vi "Manual CV-K237_V1.2.vi"() -> ()   [LabVIEW 2009]
uses:
  <vilib>/xml/Close Reference(Node).vi
  subVIs/CMSFPIX_LV80.llb/Keith 237 Operate/Standby.vi
  <vilib>/Utility/file.llb/Write To Spreadsheet File (string).vi
  <vilib>/Utility/file.llb/Write To Spreadsheet File (DBL).vi
  <vilib>/xml/NI_XML.lvlib
panel:
  in  "Stop Loop":bool
  in  "Emergency Stop":bool
  in  "Set Lower Voltage Limit":i32=-1
  in  "Bias Loop":bool
  out "Bias":dbl=5.0
  out "Compliance Level":dbl
  out "Compliance":bool
  out "Compliance":dbl=1e-09
  out "Secondary Parameter":u16(ring) items=["None", "Cs", "Cp", "Ls", "Lp", "Rs", "Rp", "DF", "Q", "Z", "Y", "Phase", "ESR", "Gp", "Xs", "Bp"]
  out "Primary Parameter":u16(ring)=2 items=["AUTO", "Cs", "Cp", "Ls", "Lp", "Rs", "Rp", "DF", "Q", "Z", "Y", "Phase", "ESR", "Gp", "Xs", "Bp"]
  out "Voltage Level":dbl=0.15
  out "Secondary Graph":cluster{"Y":dbl[], "Y":dbl[]}[](graph) caption="DF"
  out "Number of Averages":dbl=1.0
  out "Frequency":dbl=1000.0
  out "Time Delay mS":dbl=1000.0
  in  "Voltage Start":dbl
  out "Running?":bool
  in  "Device ID":string
  in  "Halt Program":bool
  in  "error in (no error)":errorcluster
  out "error out":errorcluster
  in  "Voltage Steps":dbl=2.0
  in  "Set Upper Voltage Limit":i32=10
  out "Primary Graph":cluster{"Y":dbl[], "Y":dbl[]}[](graph) caption="Cp"
  out "Initialize":string
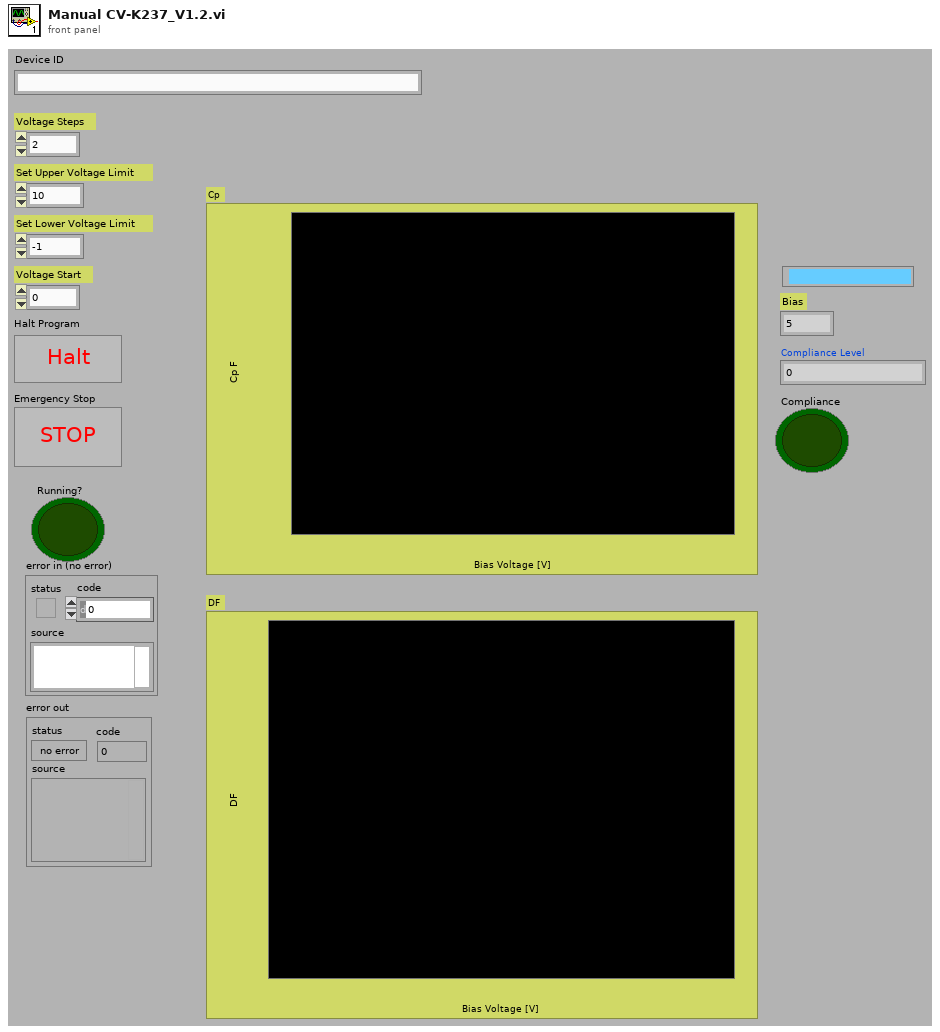
[diagram p1: front panel]
types:
  T1 = enum16{"open", "replace", "create", "open or create", "replace or create", "replace or create with confirmation"}
  T2 = cluster{"error":bool, "code":i32, "source":string}
  T3 = typedef "Semaphore RefNum" = refnum<k1>
  T4 = cluster{"error":bool, "code":i8, "source":string}
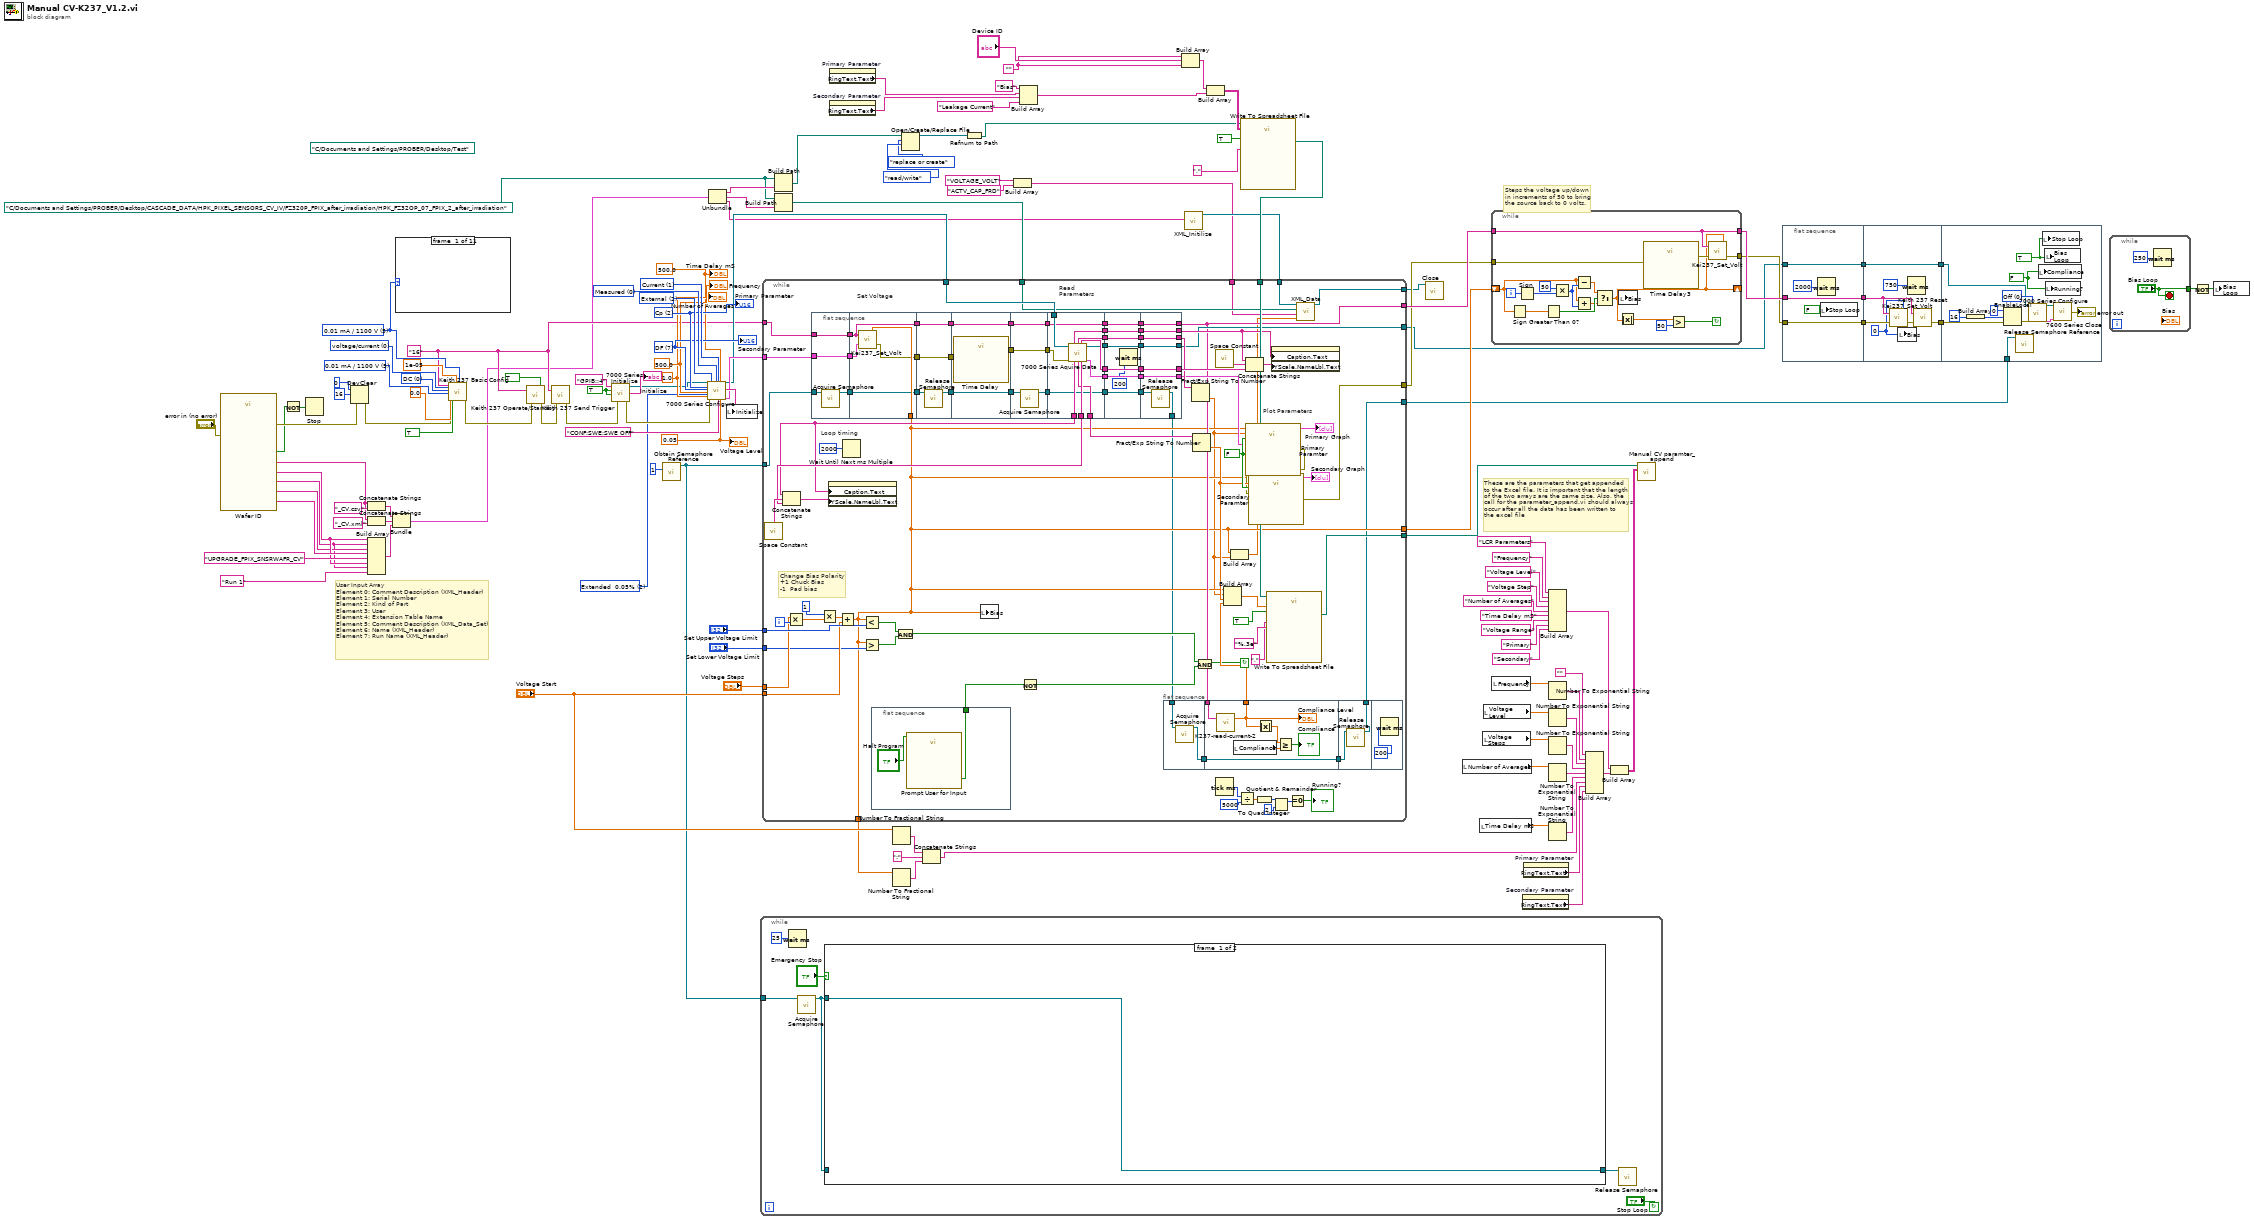
[diagram p0: block diagram]
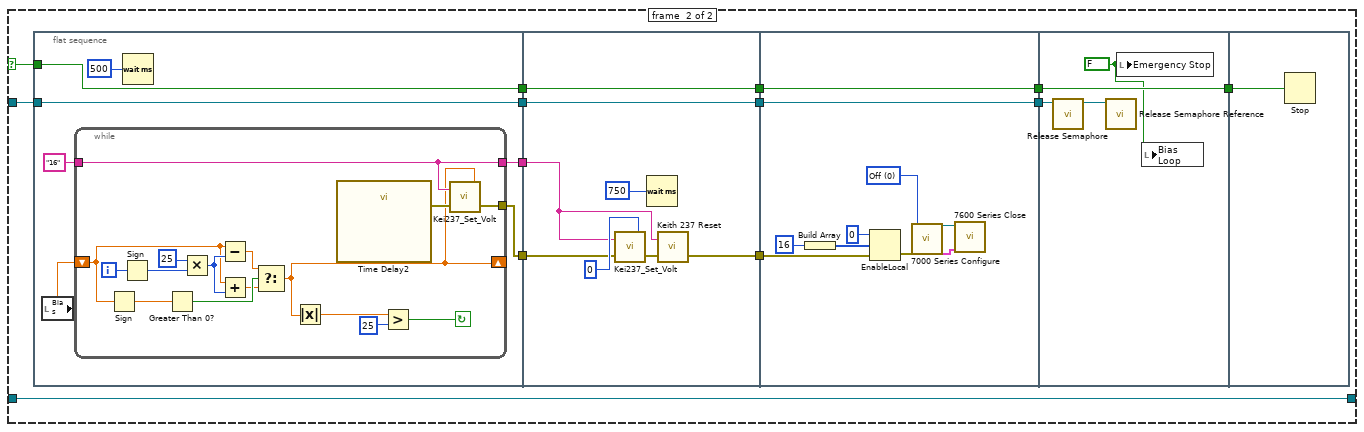
[diagram p2: hidden frame]
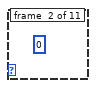
[diagram p3: hidden frame]
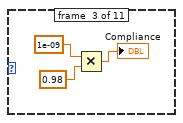
[diagram p4: hidden frame]
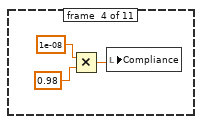
[diagram p5: hidden frame]
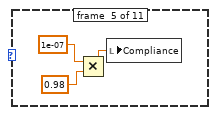
[diagram p6: hidden frame]
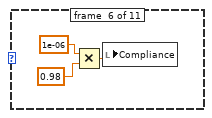
[diagram p7: hidden frame]
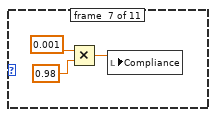
[diagram p8: hidden frame]
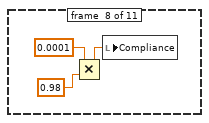
[diagram p9: hidden frame]
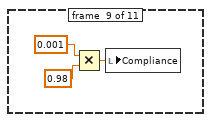
[diagram p10: hidden frame]
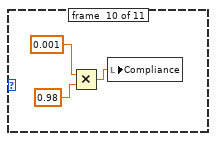
[diagram p11: hidden frame]
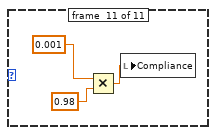
[diagram p12: hidden frame]
diagram:
  (unwired) path "C:/Documents and Settings/PROBER/Desktop/Test" ("base path")
  w87 = u16 2 items=["Basic        0.5%", "Enhanced 0.25%", "Extended  0.05%"] ("Measurement Accuracy")
  w70 = ""
  w19 = path "C:/Documents and Settings/PROBER/Desktop/CASCADE_DATA/HPK_PIXEL_SENSORS_CV_IV/FZ320P_FPIX_after_irradiation/HPK_FZ32OP_07_FPIX_2_after_irradiation" ("base path")
  w44 = u16 5 items=["auto / auto", "1 nA / 1.1 V", "10 nA / 11 V", "100 nA / 110 V", "0.001 mA / 1100 V", "0.01 mA / 1100 V", "0.1 mA / 1100 V", "1 mA / 1100 V", "10 mA / 1100 V", "100 mA / 1100 V"] ("compliance/\nmeasurement range (auto:0)")
  w107 = u16 5 items=["auto / auto", "1 nA / 1.1 V", "10 nA / 11 V", "100 nA / 110 V", "0.001 mA / 1100 V", "0.01 mA / 1100 V", "0.1 mA / 1100 V", "1 mA / 1100 V", "10 mA / 1100 V", "100 mA / 1100 V"] ("source range\nI source / V source (auto:0)")
  w112 = u16 0 items=["voltage/current", "current/voltage"] ("source/measure (V/I:0)")
  w113 = u16 0 items=["DC", "sweep"] ("function (DC:0)")
  w40 = "16" ("GPIB address")
  w115 = 500.0 ("Time Delay mS")
  w117 = TRUE ("reset")
  w69 = 0.05 ("Voltage Level")
  w122 = 1.0 ("Number of Averages")
  w123 = 500.0 ("Frequency")
  w124 = u16 7 items=["None", "Cs", "Cp", "Ls", "Lp", "Rs", "Rp", "DF", "Q", "Z", "Y", "Phase", "ESR", "Gp", "Xs", "Bp"] ("Secondary Parameter")
  w125 = u16 2 items=["AUTO", "Cs", "Cp", "Ls", "Lp", "Rs", "Rp", "DF", "Q", "Z", "Y", "Phase", "ESR", "Gp", "Xs", "Bp"] ("Primary Parameter")
  w126 = u16 1 items=["Voltage", "Current"] ("Signal Type")
  w127 = u16 0 items=["Measured", "Deviation", "% Deviation", "No Display"] ("Display")
  w128 = u16 2 items=["Off", "Internal", "External"] ("Bias")
  # "User Input Array\nElement 0: Comment Description (XML_Header)\nElement 1: Serial Number\nElement 2: Kind of Part\nElement 3: User\nElement 4: Extension Table Name\nElement 5: Comment Description (XML_Data_Set)\nElement 6: Name (XML_Header)\nElement 7: Run Name (XML_Header)"
  # "These are the parameters that get appended\nto the Excel file. It is important that the length\nof the two arrays are the same size. Also, the\ncall for the parameter_append.vi should always\noccur after all the data has been written to\nthe excel file"
  # "Steps the voltage up/down\nin increments of 50 to bring\nthe source back to 0 volts."
  n1 = call "Wafer ID"("error in (no error)"="error in (no error)") -> ("Test Name"=w7:string, "User"=w6:string, "Kind of Part"=w3:string, "Part Name"=w2:string, "Comment Description"=w4:string, "OK"=w93:bool, "error out"=w98:errorcluster)  [unwired: 11 in, 1 out]
  n2 = Not(x=w93) -> (.not. x?=w92:bool)
  n3 = Stop(stop? (T)=w92) -> ()
  n4 = DevClear(2:w98, 3:i16 16 ("address"), 4:0) -> (0:w103:errorcluster)  [unwired: 1 out]
  n5 = Concatenate Strings(w7, "_CV.csv" ("string")) -> (w24:string)
  n6 = Concatenate Strings(w7, "_CV.xml" ("string")) -> (w23:string)
  n7 = Build Array(w4, w2, w3, w6, "UPGRADE_FPIX_SNSRWAFR_CV", w4, w2, "Run 1" ("element")) -> (w13:string[])
  n8 = Bundle(w24, w23, w13) -> (w20:cluster{string, string, string[]})  [unwired: 1 in]
  n9 = case shown="1" w44 {
    frame #0 {
    }
    frame #1 {
      (unwired) 0
    }
    frame #2 {
      n10 = Multiply(x=1e-09, y=0.98) -> (x*y=→"Compliance":dbl)
    }
    frame #3 {
      n11 = Multiply(x=1e-08, y=0.98) -> (x*y=w133:dbl)
      n12 = local write "Compliance"(w133) -> ()
    }
    frame #4 {
      n13 = Multiply(x=1e-07, y=0.98) -> (x*y=w136:dbl)
      n14 = local write "Compliance"(w136) -> ()
    }
    frame #5 {
      n15 = Multiply(x=1e-06, y=0.98) -> (x*y=w139:dbl)
      n16 = local write "Compliance"(w139) -> ()
    }
    frame #6 {
      n17 = Multiply(x=0.001, y=0.98) -> (x*y=w143:dbl)
      n18 = local write "Compliance"(w143) -> ()
    }
    frame #7 {
      n19 = Multiply(x=0.0001, y=0.98) -> (x*y=w145:dbl)
      n20 = local write "Compliance"(w145) -> ()
    }
    frame #8 {
      n21 = Multiply(x=0.001, y=0.98) -> (x*y=w149:dbl)
      n22 = local write "Compliance"(w149) -> ()
    }
    frame #9 {
      n23 = Multiply(x=0.001, y=0.98) -> (x*y=w151:dbl)
      n24 = local write "Compliance"(w151) -> ()
    }
    frame #10 {
      n25 = Multiply(x=0.001, y=0.98) -> (x*y=w154:dbl)
      n26 = local write "Compliance"(w154) -> ()
    }
  }
  n27 = call "Keith 237 Basic Config.vi"("GPIB address"=w40, "source/measure (V/I:0)"=w112, "function (DC:0)"=w113, "source range\nI source / V source (auto:0)"=w107, "source level"=0.0, "error in"=w103, "1100 V range (disabled:F)"=TRUE, "current \ncompliance level"=1e-05 ("current \ncompliance level"), "compliance/\nmeasurement range (auto:0)"=w44) -> ("error out"=w110:T2)  [unwired: 10 in]
  n28 = call "Keith 237 Operate/Standby.vi"("source"=TRUE, "error in"=w110, "GPIB address"=w40) -> ("error out"=w108:T2)
  n29 = call "Keith 237 Send Trigger.vi"("GPIB address"=w40, "error in"=w108) -> ("error out"=w102:T2)
  n30 = call "7000 Series Initialize.vi"("error in (no error)"=w102, "reset"=w117, "ID query"=w117, "instrument descriptor"="GPIB::4") -> ("error out"=w129:errorcluster, "Identification"=→"Initialize":string, "VISA session"=w118:refnum<visa-resource-name>)
  n31 = call <vilib>:"Obtain Semaphore Reference.vi"("size (1)"=1) -> ("semaphore"=w10:T3)  [unwired: 4 in, 2 out]
  n32 = call "7000 Series Configure.vi"("inst handle in"=w118, "Primary Parameter"=w125, "Secondary Parameter"=w124, "Frequency"=w123, "Measurement Accuracy"=w87, "Number of Averages"=w122, "error in"=w129, "Bias"=w128, "Display"=w127, "Signal Type"=w126, "Optional"="CONF:SWE:SWE OFF", "Time Delay mS"=w115, "Voltage Level"=w69) -> ("inst handle out"=w100:refnum<visa-resource-name>, "Identification"=w119:string, "error out"=w101:T4)  [unwired: 12 in]
  n33 = Unbundle(w20) -> (w22:string, w21:string, w12:string[])
  n34 = local write "Initialize"(w119) -> ()
  n35 = while {
    tunnel: w10 -> [w161]
    stop <- "Stop Loop" continue-if-true
    n36 = Wait (ms)(milliseconds to wait=25) -> ()  [unwired: 1 out]
    n37 = call <vilib>:"Acquire Semaphore.vi"("semaphore"=w161) -> ("semaphore out"=w158:T3)  [unwired: 4 in, 2 out]
    n38 = case shown="True" "Emergency Stop" {
      selector: "Emergency Stop" -> [_ w175]
      tunnel: w158 -> [w163 w176]
      tunnel: [w163 w173] -> w159
      tunnel: w158 -> [_ w173]
      frame #0 {
      }
      frame #1 {
        n39 = flat-sequence {
          tunnel: [w182] -> w172
          tunnel: w176 -> [w182]
          tunnel: [w181] -> w171
          tunnel: w175 -> [w181]
          tunnel: [w180] -> w166
          tunnel: [w178] -> w165
          tunnel: w172 -> [w207]
          tunnel: [w207] -> w170
          tunnel: w171 -> [w206]
          tunnel: [w206] -> w168
          tunnel: w166 -> [w202]
          tunnel: w165 -> [w201]
          tunnel: [w200] -> w164
          tunnel: w170 -> [w217]
          tunnel: [w217] -> w169
          tunnel: w168 -> [w216]
          tunnel: [w216] -> w167
          tunnel: w164 -> [w208]
          tunnel: w169 -> [w219]
          tunnel: w167 -> [w221]
          tunnel: [w221] -> w174
          tunnel: w174 -> [w222]
          frame #0 {
            n40 = local read "Bias"() -> (w177:dbl)
            n41 = while {
              tunnel: [w199] -> w180
              tunnel: "16" ("GPIB address") -> [w194]
              tunnel: [w194] -> w178
              shift-right: [w184] -> _
              shift-left: w177 -> [w187]
              i -> [w186]
              stop <- w196 continue-if-true
              n42 = Sign(1:w187) -> (0:w193:dbl)
              n43 = Sign(1:w186) -> (0:w185:i32)
              n44 = Greater Than 0?(x=w193) -> (x > 0?=w192:bool)
              n45 = Multiply(x=25, y=w185) -> (x*y=w191:i32)
              n46 = Subtract(x=w187, y=w191) -> (x-y=w190:dbl)
              n47 = Add(x=w187, y=w191) -> (x+y=w189:dbl)
              n48 = Select(t=w190, s=w192, f=w189) -> (s? t:f=w184:dbl)
              n49 = Absolute Value(x=w184) -> (abs(x)=w188:dbl)
              n50 = call "Time Delay2"() -> ("error out"=w195:errorcluster)  [unwired: 11 in]
              n51 = Greater?(x=w188, y=25) -> (0:w196:bool)
              n52 = call "Kei237_Set_Volt.vi"("Voltage"=w184, "error in"=w195, "GPIB"=w194) -> ("error out"=w199:errorcluster)
            }
            n53 = Wait (ms)(milliseconds to wait=500) -> ()  [unwired: 1 out]
          }
          frame #1 {
            n54 = call "Kei237_Set_Volt.vi"("Voltage"=0, "error in"=w202, "GPIB"=w201) -> ("error out"=w203:errorcluster)
            n55 = Wait (ms)(milliseconds to wait=750) -> ()  [unwired: 1 out]
            n56 = call "Keith 237 Reset.vi"("GPIB address"=w201, "error in"=w203) -> ("error out"=w200:T2)
          }
          frame #2 {
            w214 = u16 0 items=["Off", "Internal", "External"] ("Bias")
            n57 = Build Array(16) -> (w215:i32[])
            n58 = EnableLocal(2:w208, 3:w215, 4:0) -> (0:w211:errorcluster)  [unwired: 1 out]
            n59 = call "7000 Series Configure.vi"("error in"=w211, "Bias"=w214) -> ("inst handle out"=w212:refnum<visa-resource-name>, "error out"=w213:T4)  [unwired: 23 in, 1 out]
            n60 = call "7600 Series Close.vi"("error in (no error)"=w213, "VISA session"=w212) -> ()  [unwired: 2 in, 1 out]
          }
          frame #3 {
            w220 = FALSE ("Emergency Stop")
            n61 = call <vilib>:"Release Semaphore.vi"("semaphore"=w219) -> ("semaphore out"=w218:T3)  [unwired: 5 in, 1 out]
            n62 = call <vilib>:"Release Semaphore Reference.vi"("semaphore"=w218) -> ()  [unwired: 9 in, 2 out]
            n63 = local write "Emergency Stop"(w220) -> ()
            n64 = local write "Bias Loop"(w220) -> ()
          }
          frame #4 {
            n65 = Stop(stop? (T)=w222) -> ()
          }
        }
      }
    }
    n66 = call <vilib>:"Release Semaphore.vi"("semaphore"=w159) -> ()  [unwired: 5 in, 2 out]
  }
  n67 = Build Path(base path=w19, name or relative path=w22) -> (appended path=w85:path)
  n68 = Build Path(base path=w19, name or relative path=w21) -> (appended path=w17:path)
  n69 = property on="Secondary Parameter" class="Ring (strict)"() -> ("RingText.Text"=w51:string)  [unwired: 2 in, 2 out]
  n70 = property on="Primary Parameter" class="Ring (strict)"() -> ("RingText.Text"=w52:string)  [unwired: 2 in, 2 out]
  n71 = Number To Fractional String(number="Voltage Start") -> (F-format string=w45:string)  [unwired: 3 in]
  n72 = Open/Create/Replace File(file path (use dialog)=w85, operation (0:open)=T1."replace or create", access (0:read/write)=enum16{"read/write", "read-only", "write-only"}."read/write") -> (refnum out=w80:refnum<file>)  [unwired: 1 in, 4 out]
  n73 = Refnum to Path(1:w80) -> (0:w79:path)
  n74 = Build Array("VOLTAGE_VOLT", "ACTV_CAP_FRD") -> (w14:string[])
  n75 = Build Array("Bias", w52, w51, "Leakage Current" ("element")) -> (w90:string[])
  n76 = Build Array(w70, "Device ID", w70) -> (w89:string[])
  n77 = call "XML_Initilize.vi"("User Input"=w12) -> ("DOM document out"=w18:refnum<k20>)  [unwired: 10 in]
  n78 = Build Array(w89, w90) -> (w88:string[][])
  n79 = call-poly <vilib>:"Write To Spreadsheet File.vi"("delimiter (\\t)"=",", "append to file? (new file:F)"=TRUE, "2D data"=w88, "file path (dialog if empty)"=w79) -> ("new file path (Not A Path if cancelled)"=w78:path)  [unwired: 3 in, 1 out]
  n80 = while {
    tunnel: w40 -> [w285]
    tunnel: w101 -> [w284]
    tunnel: "Set Upper Voltage Limit" -> [w299]
    tunnel: "Voltage Steps" -> [w288]
    tunnel: w100 -> [w283]
    tunnel: [w287] -> w37
    tunnel: w78 -> [w309]
    tunnel: [w274] -> w39
    tunnel: "Voltage Start" -> [w289]
    tunnel: [w290] -> w73
    tunnel: [w255] -> w47
    tunnel: [w255] -> w38
    tunnel: [w275] -> w32
    tunnel: "Set Lower Voltage Limit" -> [w259]
    tunnel: w18 -> [w258]
    tunnel: w17 -> [w257]
    tunnel: w14 -> [w256]
    tunnel: w10 -> [w228]
    tunnel: [w224] -> w9
    tunnel: [w223] -> w8
    i -> [w314]
    stop <- w265 continue-if-true
    w296 = FALSE ("Reset")
    # "Read \nParameters"
    # "Set Voltage"
    # "Change Bias Polarity\n+1 Chuck Bias\n-1  Pad bias"
    # "Loop timing"
    # "Plot Parameters"
    n81 = call <vilib>:"Space Constant.vi"() -> ("String"=w292:string)
    n82 = Concatenate Strings(w276, w292, w278) -> (w291:string)
    n83 = Multiply(x=w288, y=w314) -> (x*y=w312:dbl)
    n84 = flat-sequence {
      tunnel: w285 -> [w328]
      tunnel: w284 -> [w329]
      tunnel: [w329] -> w237
      tunnel: [w328] -> w236
      tunnel: [w327] -> w234
      tunnel: w228 -> [w326]
      tunnel: w255 -> [w333]
      tunnel: [w332] -> w241
      tunnel: [w331] -> w239
      tunnel: w237 -> [w334]
      tunnel: w236 -> [w331]
      tunnel: [w330] -> w235
      tunnel: w234 -> [w330]
      tunnel: w241 -> [w338]
      tunnel: [w338] -> w240
      tunnel: w239 -> [w337]
      tunnel: [w337] -> w238
      tunnel: w235 -> [w336]
      tunnel: [w335] -> w232
      tunnel: w240 -> [w342]
      tunnel: [w341] -> w245
      tunnel: [w340] -> w243
      tunnel: w238 -> [w340]
      tunnel: [w339] -> w233
      tunnel: w232 -> [w339]
      tunnel: w245 -> [w346]
      tunnel: [w346] -> w244
      tunnel: w243 -> [w345]
      tunnel: [w345] -> w242
      tunnel: w233 -> [w344]
      tunnel: [w343] -> w229
      tunnel: w244 -> [w358]
      tunnel: w283 -> [w357]
      tunnel: [w352] -> w276
      tunnel: [w351] -> w278
      tunnel: [w350] -> w277
      tunnel: w242 -> [w348]
      tunnel: [w356] -> w272
      tunnel: [w355] -> w271
      tunnel: [w354] -> w270
      tunnel: [w353] -> w269
      tunnel: [w349] -> w268
      tunnel: [w348] -> w267
      tunnel: [w347] -> w230
      tunnel: w229 -> [w347]
      tunnel: w272 -> [w366]
      tunnel: w271 -> [w365]
      tunnel: w270 -> [w364]
      tunnel: w269 -> [w363]
      tunnel: w268 -> [w362]
      tunnel: w267 -> [w361]
      tunnel: [w366] -> w251
      tunnel: [w365] -> w250
      tunnel: [w364] -> w249
      tunnel: [w363] -> w248
      tunnel: [w362] -> w247
      tunnel: [w361] -> w246
      tunnel: [w359] -> w231
      tunnel: w230 -> [w359]
      tunnel: [w369] -> w274
      tunnel: [w370] -> w275
      tunnel: [w371] -> w279
      tunnel: [w372] -> w280
      tunnel: [w373] -> w282
      tunnel: [w374] -> w281
      tunnel: w251 -> [w374]
      tunnel: w250 -> [w373]
      tunnel: w249 -> [w372]
      tunnel: w248 -> [w371]
      tunnel: w247 -> [w370]
      tunnel: w246 -> [w369]
      tunnel: w231 -> [w368]
      tunnel: [w367] -> w227
      frame #0 {
        n85 = call <vilib>:"Acquire Semaphore.vi"("semaphore"=w326) -> ("semaphore out"=w327:T3)  [unwired: 4 in, 2 out]
      }
      frame #1 {
        n86 = call "Kei237_Set_Volt.vi"("Voltage"=w333, "error in"=w334, "GPIB"=w331) -> ("error out"=w332:errorcluster)
      }
      frame #2 {
        n87 = call <vilib>:"Release Semaphore.vi"("semaphore"=w336) -> ("semaphore out"=w335:T3)  [unwired: 5 in, 1 out]
      }
      frame #3 {
        n88 = call "Time Delay"("error in (no error)"=w342) -> ("error out"=w341:errorcluster)  [unwired: 10 in]
      }
      frame #4 {
        n89 = call <vilib>:"Acquire Semaphore.vi"("semaphore"=w344) -> ("semaphore out"=w343:T3)  [unwired: 4 in, 2 out]
      }
      frame #5 {
        n90 = call "7000 Series Aquire Data.vi"("inst handle in"=w357, "error in"=w358) -> ("Primary"=w356:string, "Primary Value"=w354:string, "Primary Unit"=w355:string, "inst handle out"=w349:refnum<visa-resource-name>, "Secondary"=w352:string, "Secondary Value"=w350:string, "Secondary Unit"=w351:string, "error out"=w353:T4)  [unwired: 5 in, 1 out]
      }
      frame #6 {
        n91 = Wait (ms)(milliseconds to wait=200) -> ()  [unwired: 1 out]
      }
      frame #7 {
        n92 = call <vilib>:"Release Semaphore.vi"("semaphore"=w368) -> ("semaphore out"=w367:T3)  [unwired: 5 in, 1 out]
      }
    }
    n93 = Multiply(x=1, y=w312) -> (x*y=w300:dbl)
    n94 = property on="Secondary Parameter" class="XYGraph (strict)"("Caption.Text"=w276, "YScale.NameLbl.Text"=w291) -> ()  [unwired: 2 in, 2 out]
    n95 = Add(x=w300, y=w289) -> (x+y=w255:dbl)
    n96 = Wait Until Next ms Multiple(millisecond multiple=u32 2000) -> ()  [unwired: 1 out]
    n97 = Less?(x=w255, y=w299) -> (x < y?=w262:bool)
    n98 = Greater?(x=w255, y=w259) -> (0:w261:bool)
    n99 = flat-sequence {
      tunnel: [w375] -> w263
      frame #0 {
        n100 = call "Prompt User for Input"("Enable"="Halt Program") -> ("Yes"=w375:bool)  [unwired: 17 in, 1 out]
      }
    }
    n101 = And(x=w262, y=w261) -> (x .and. y?=w260:bool)
    n102 = local write "Bias"(w255) -> ()
    n103 = Not(x=w263) -> (.not. x?=w264:bool)
    n104 = flat-sequence {
      tunnel: w227 -> [w316]
      tunnel: [w315] -> w225
      tunnel: w274 -> [w320]
      tunnel: [w318] -> w266
      tunnel: [w317] -> w226
      tunnel: w225 -> [w317]
      tunnel: w226 -> [w324]
      tunnel: [w323] -> w223
      frame #0 {
        n105 = call <vilib>:"Acquire Semaphore.vi"("semaphore"=w316) -> ("semaphore out"=w315:T3)  [unwired: 4 in, 2 out]
      }
      frame #1 {
        n106 = call "K237-read-current-2.vi"("GPIB"=w320) -> ("Current"=w318:dbl)  [unwired: 1 in, 1 out]
        "Compliance Level" <- w318
        n107 = local read "Compliance"() -> (w322:dbl)
        n108 = Absolute Value(x=w318) -> (abs(x)=w319:dbl)
        n109 = Greater Or Equal?(x=w319, y=w322) -> (x >= y?=→"Compliance":bool)
      }
      frame #2 {
        n110 = call <vilib>:"Release Semaphore.vi"("semaphore"=w324) -> ("semaphore out"=w323:T3)  [unwired: 5 in, 1 out]
      }
      frame #3 {
        n111 = Wait (ms)(milliseconds to wait=200) -> ()  [unwired: 1 out]
      }
    }
    n112 = Fract/Exp String To Number(string=w280) -> (number=w254:dbl)  [unwired: 3 in, 1 out]
    n113 = Fract/Exp String To Number(string=w277) -> (number=w295:dbl)  [unwired: 3 in, 1 out]
    n114 = And(x=w260, y=w264) -> (x .and. y?=w265:bool)
    n115 = Tick Count (ms)() -> (millisecond timer value=w305:u32)
    n116 = call <vilib>:"Space Constant.vi"() -> ("String"=w293:string)
    n117 = Build Array(w255, w254, w295, w266) -> (w253:dbl[])
    n118 = Build Array(w255, w254) -> (w252:dbl[])
    n119 = Divide(x=w305, y=5000) -> (x/y=w303:dbl)
    n120 = call "Primary Paramter"("error in (no error)"=w279, "Reset"=w296, "Y Input"=w254, "X Input"=w255) -> ("error out"=w286:errorcluster, "XY Graph"=→"Primary Graph":cluster{"Y":dbl[], "Y":dbl[]}[])  [unwired: 1 in, 5 out]
    n121 = Concatenate Strings(w281, w293, w282) -> (w294:string)
    n122 = call "Secondary Paramter"("error in (no error)"=w286, "Reset"=w296, "Y Input"=w295, "X Input"=w255) -> ("error out"=w287:errorcluster, "XY Graph"=→"Secondary Graph":cluster{"Y":dbl[], "Y":dbl[]}[])  [unwired: 1 in, 5 out]
    n123 = To Quad Integer(1:w303) -> (0:w302:i64)
    n124 = call-poly <vilib>:"Write To Spreadsheet File.vi"("delimiter (\\t)"=",", "format (%.3f)"="%.3e" ("file format"), "append to file? (new file:F)"=TRUE, "1D data"=w253, "file path (dialog if empty)"=w309) -> ("new file path (Not A Path if cancelled)"=w290:path)  [unwired: 2 in, 1 out]
    n125 = property on="Primary Parameter" class="XYGraph (strict)"("Caption.Text"=w281, "YScale.NameLbl.Text"=w294) -> ()  [unwired: 2 in, 2 out]
    n126 = Quotient & Remainder(x=w302, y=2) -> (x-y*floor(x/y)=w306:i64)  [unwired: 1 out]
    n127 = Equal To 0?(x=w306) -> (x = 0?=→"Running?":bool)
    n128 = call "XML_Data.vi"("Data Input Array"=w252, "Data Tag Names Array"=w256, "XML File Path"=w257, "DOM document in"=w258) -> ("DOM document out"=w224:refnum<k20>)  [unwired: 6 in, 1 out]
  }
  n129 = Number To Fractional String(number=w47) -> (F-format string=w49:string)  [unwired: 3 in]
  n130 = Concatenate Strings(w45, ":", w49) -> (w46:string)
  n131 = call-poly <vilib>:"Close.vi"("node"=w9) -> ()  [unwired: 8 in, 1 out]
  n132 = local read "Number of Averages"() -> (w82:dbl)
  n133 = local read "Time Delay mS"() -> (w81:dbl)
  n134 = local read "Voltage Steps"() -> (w83:dbl)
  n135 = local read "Voltage Level"() -> (w68:dbl)
  n136 = while {
    tunnel: [w393] -> w35
    tunnel: w37 -> [w388]
    tunnel: w39 -> [w387]
    tunnel: [w387] -> w36
    shift-right: [w377] -> _
    shift-left: w38 -> [w380]
    i -> [w379]
    stop <- w390 continue-if-true
    n137 = Sign(1:w380) -> (0:w386:dbl)
    n138 = Sign(1:w379) -> (0:w378:i32)
    n139 = Greater Than 0?(x=w386) -> (x > 0?=w385:bool)
    n140 = Multiply(x=50, y=w378) -> (x*y=w384:i32)
    n141 = Subtract(x=w380, y=w384) -> (x-y=w383:dbl)
    n142 = Add(x=w380, y=w384) -> (x+y=w382:dbl)
    n143 = Select(t=w383, s=w385, f=w382) -> (s? t:f=w377:dbl)
    n144 = local write "Bias"(w377) -> ()
    n145 = Absolute Value(x=w377) -> (abs(x)=w381:dbl)
    n146 = call "Time Delay3"("error in (no error)"=w388) -> ("error out"=w389:errorcluster)  [unwired: 10 in]
    n147 = Greater?(x=w381, y=50) -> (0:w390:bool)
    n148 = call "Kei237_Set_Volt.vi"("Voltage"=w377, "error in"=w389, "GPIB"=w387) -> ("error out"=w393:errorcluster)
  }
  n149 = local read "Frequency"() -> (w72:dbl)
  n150 = property on="Secondary Parameter" class="Ring (strict)"() -> ("RingText.Text"=w66:string)  [unwired: 2 in, 2 out]
  n151 = property on="Primary Parameter" class="Ring (strict)"() -> ("RingText.Text"=w67:string)  [unwired: 2 in, 2 out]
  n152 = Build Array("LCR Parameters" ("element"), "Frequency", "Voltage Level", "Voltage Step", "Number of Averages", "Time Delay mS", "Voltage Range", "Primary", "Secondary") -> (w55:string[])
  n153 = Number To Exponential String(number=w72) -> (E-format string=w77:string)  [unwired: 3 in]
  n154 = Number To Exponential String(number=w68) -> (E-format string=w76:string)  [unwired: 3 in]
  n155 = Number To Exponential String(number=w83) -> (E-format string=w63:string)  [unwired: 3 in]
  n156 = Number To Exponential String(number=w82) -> (E-format string=w64:string)  [unwired: 3 in]
  n157 = Number To Exponential String(number=w81) -> (E-format string=w65:string)  [unwired: 3 in]
  n158 = Build Array("", w77, w76, w63, w64, w65, w46, w67, w66) -> (w75:string[])
  n159 = Build Array(w55, w75) -> (w74:string[][])
  n160 = call "Manual CV paramter_append.vi"("Array"=w74, "Path"=w73) -> ()  [unwired: 9 in, 1 out]
  n161 = flat-sequence {
    tunnel: w36 -> [w397]
    tunnel: w35 -> [w398]
    tunnel: [w398] -> w43
    tunnel: [w397] -> w42
    tunnel: w32 -> [w395]
    tunnel: [w395] -> w30
    tunnel: w43 -> [w405]
    tunnel: w42 -> [w403]
    tunnel: [w402] -> w41
    tunnel: [w399] -> w31
    tunnel: w30 -> [w399]
    tunnel: w41 -> [w411]
    tunnel: w31 -> [w408]
    tunnel: w8 -> [w406]
    frame #0 {
      n162 = Wait (ms)(milliseconds to wait=2000) -> ()  [unwired: 1 out]
      n163 = local write "Stop Loop"(FALSE ("Boolean")) -> ()
    }
    frame #1 {
      w400 = 0
      n164 = call "Kei237_Set_Volt.vi"("Voltage"=w400, "error in"=w405, "GPIB"=w403) -> ("error out"=w404:errorcluster)
      n165 = local write "Bias"(w400) -> ()
      n166 = Wait (ms)(milliseconds to wait=750) -> ()  [unwired: 1 out]
      n167 = call "Keith 237 Reset.vi"("GPIB address"=w403, "error in"=w404) -> ("error out"=w402:T2)
    }
    frame #2 {
      w407 = TRUE
      w409 = FALSE
      w413 = u16 0 items=["Off", "Internal", "External"] ("Bias")
      n168 = Build Array(16) -> (w410:i32[])
      n169 = EnableLocal(2:w411, 3:w410, 4:0) -> (0:w416:errorcluster)  [unwired: 1 out]
      n170 = call <vilib>:"Release Semaphore Reference.vi"("semaphore"=w406) -> ()  [unwired: 9 in, 2 out]
      n171 = call "7000 Series Configure.vi"("inst handle in"=w408, "error in"=w416, "Bias"=w413) -> ("inst handle out"=w415:refnum<visa-resource-name>, "error out"=w414:T4)  [unwired: 22 in, 1 out]
      n172 = local write "Compliance"(w409) -> ()
      n173 = local write "Stop Loop"(w407) -> ()
      n174 = local write "Bias Loop"(w407) -> ()
      n175 = local write "Running?"(w409) -> ()
      n176 = call "7600 Series Close.vi"("error in (no error)"=w414, "VISA session"=w415) -> ("error out"=→"error out":errorcluster)  [unwired: 2 in]
    }
  }
  n177 = while {
    tunnel: ["Bias Loop"] -> w34
    stop <- "Bias Loop" stop-if-true
    n178 = Wait (ms)(milliseconds to wait=250) -> ()  [unwired: 1 out]
  }
  n179 = Not(x=w34) -> (.not. x?=w33:bool)
  n180 = local write "Bias Loop"(w33) -> ()
  "Time Delay mS" <- w115
  "Frequency" <- w123
  "Number of Averages" <- w122
  "Voltage Level" <- w69
  "Primary Parameter" <- w125
  "Secondary Parameter" <- w124
